vi "RIOSuperSampleMaster.vi"() -> ()   [LabVIEW 2012]
doc: "A sample master that can be run on the computer or RIO"
panel:
  out "time":string
  out "Status":string
  in  "stop":bool
  # "Instructions:\n1. Run the VI\n2. Verify that you see the correct time.\n3. Press the LED button. You should see the LED reply change.\nIf you are targetting a myRIO, the LED should change as well.\n4. Debug by clicking Show Node and Show Webpage.\n5. See what is being sent back and forth by clicking Show Node and Show Webpage."
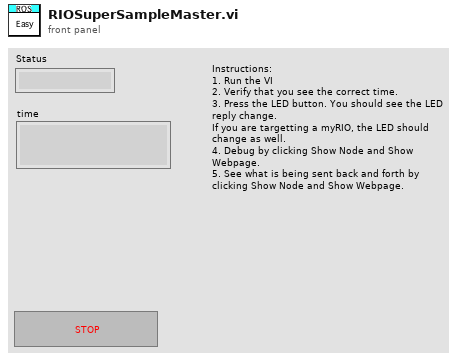
[diagram p1: front panel]
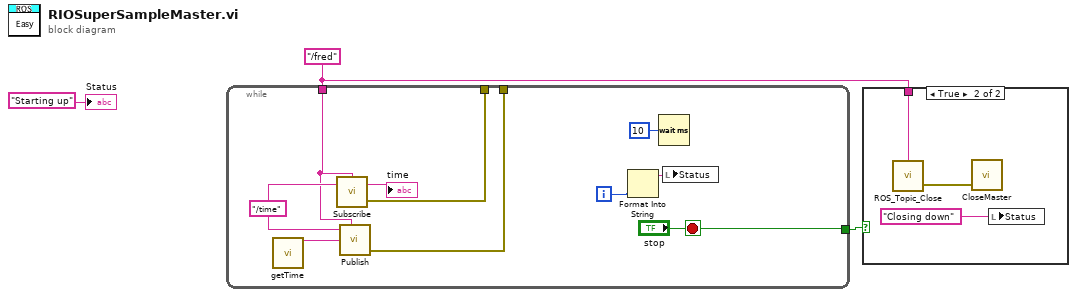
[diagram p0: block diagram]
diagram:
  w1 = "/fred" ("Topic")
  n1 = while {
    tunnel: ["stop"] -> w2
    tunnel: w1 -> [w8]
    tunnel: [w5] -> _
    tunnel: [w4] -> _
    i -> [w6]
    stop <- "stop" stop-if-true
    w9 = "/time" ("Topic")
    n2 = call <userlib>:"getTime.vi"() -> ("Current Time"=w10:string)  [unwired: 1 in]
    n3 = call <userlib>:"Subscribe.vi"("Topic"=w9, "node"=w8) -> ("error out"=w5:errorcluster, "Reply"=→"time":string)  [unwired: 1 in]
    n4 = call <userlib>:"Publish.vi"("Topic"=w9, "node"=w8, "String"=w10) -> ("error"=w4:errorcluster)  [unwired: 4 in]
    n5 = Format Into String(w6) -> (resulting string=w12:string)  [unwired: 3 in, 1 out]
    n6 = Wait (ms)(milliseconds to wait=u32 10) -> ()  [unwired: 1 out]
    n7 = local write "Status"(w12) -> ()
  }
  n8 = case shown="True" w2 {
    tunnel: w1 -> [_ w15]
    frame False {
    }
    frame True {
      n9 = call <userlib>:"ROS_Topic_Close.vi"("node"=w15) -> ("error out"=w14:errorcluster)  [unwired: 3 in]
      n10 = call <userlib>:"CloseMaster.vi"("error in (no error)"=w14) -> ()  [unwired: 2 in, 1 out]
      n11 = local write "Status"("Closing down" ("Status")) -> ()
    }
  }
  "Status" <- "Starting up" ("Status")
